vi "NR Configure Common.vi"(0 "RFmx Handle In":refnum<k21>, 1 "Selector String":string, 5 "Common Configuration":T1={"Center Frequency (Hz)"=3500000000.0, "Reference Level (dBm)"=0.0, "External Attenuation (dB)"=0.0, "Trigger Enabled"=TRUE, "Selected Ports"="", "IQ Power Edge Level (dB or dBm)"=0.0, "IQ Power Edge Source"="PXI_Trig0"} {"IQ Power Edge Level (dB or dBm)" format="%.2p"; "External Attenuation (dB)" format="%.2f"; "Reference Level (dBm)" format="%.2f"; "Center Frequency (Hz)" format="%.6p"}, 11 "error in (no error)":errorcluster) -> (4 "RFmx Handle Out":refnum<k21>, 15 "error out":errorcluster)   [LabVIEW 2019, in "RFmxNR.lvlib"]
doc: "Configures common measurement settings for the personality."
uses:
  RFmxNR.lvlib
  Common/SA Common Configuration.ctl
  <vilib>/RFmx/NR/mx/RFmxNR.llb/RFmxNR Configure IQ Power Edge Trigger.vi
  <resource>/objmgr/RFmxNR.rc
  Common/Common.lvlib
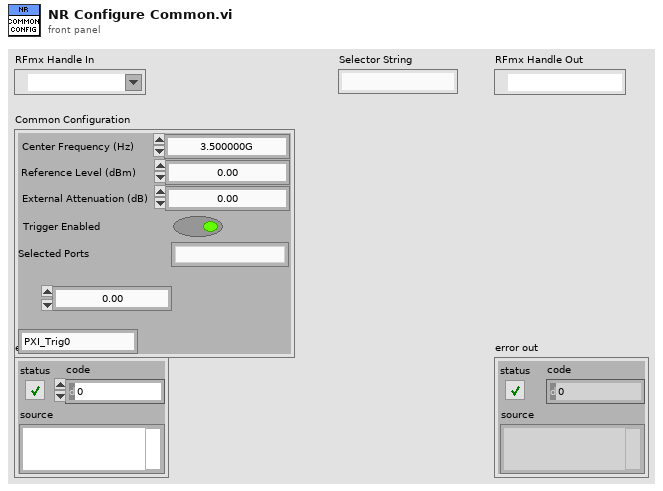
[diagram p1: front panel]
types:
  T1 = typedef "Common.lvlib/SA Common Configuration.ctl" = cluster{"Center Frequency (Hz)":dbl, "Reference Level (dBm)":dbl, "External Attenuation (dB)":dbl, "Trigger Enabled":bool, "Selected Ports":string, "IQ Power Edge Level (dB or dBm)":dbl, "IQ Power Edge Source":string}
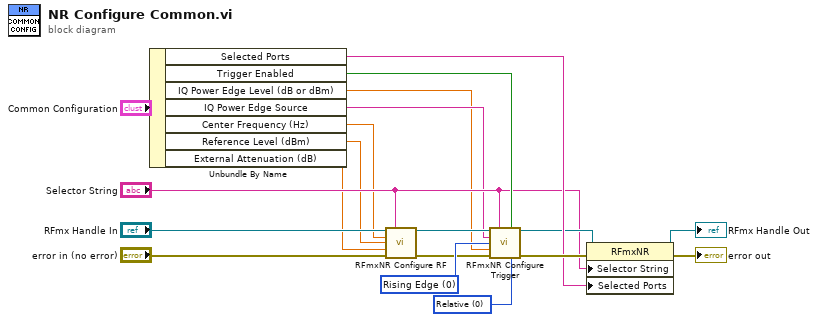
[diagram p0: block diagram]
diagram:
  w1 = 0 items=["Relative", "Absolute"] ("IQ Power Edge Level Type")
  w13 = 0 items=["Rising Edge", "Falling Edge"] ("Digital Edge")
  n1 = Unbundle By Name("Common Configuration") -> ("Selected Ports"=w12:string, "Trigger Enabled"=w16:bool, "IQ Power Edge Level (dB or dBm)"=w2:dbl, "IQ Power Edge Source"=w3:string, "Center Frequency (Hz)"=w6:dbl, "Reference Level (dBm)"=w5:dbl, "External Attenuation (dB)"=w4:dbl)
  n2 = call <vilib>:"RFmxNR Configure RF.vi"("Instrument Handle In"="RFmx Handle In", "Selector String"="Selector String", "Center Frequency (Hz)"=w6, "Reference Level"=w5, "External Attenuation (dB)"=w4, "error in (no error)"="error in (no error)") -> ("Instrument Handle Out"=w9:refnum<k21>, "error out"=w8:errorcluster)  [unwired: 8 in]
  n3 = call-poly <vilib>:"RFmxNR Configure Trigger.vi"("Instrument Handle In"=w9, "Selector String"="Selector String", "Enable Trigger?"=w16, "IQ Power Edge Source"=w3, "IQ Power Edge Slope"=w13, "IQ Power Edge Level (dB or dBm)"=w2, "error in (no error)"=w8, "IQ Power Edge Level Type"=w1) -> ("Instrument Handle Out"=w11:refnum<k21>, "error out"=w17:errorcluster)  [unwired: 6 in]
  n4 = property class="RFmxNR"(reference=w11, error in=w17, "Selector String"="Selector String", "Selected Ports"=w12) -> (reference out=→"RFmx Handle Out":refnum<k21>, error out=→"error out":errorcluster)
